vi "GetShortcut.vi"(8 "error in (no error)":errorcluster, 11 "separator item in":refnum<class "separator item.lvclass">) -> (0 "error out":errorcluster, 2 "shortcut":string, 3 "separator item out":refnum<class "separator item.lvclass">)   [LabVIEW 2009, in "separator item.lvclass"]
uses:
  separator item.lvclass
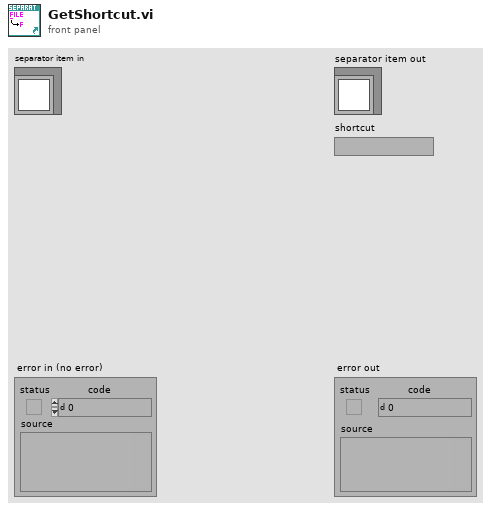
[diagram p1: front panel]
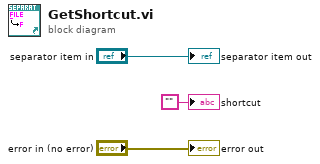
[diagram p0: block diagram]
diagram:
  "separator item out" <- "separator item in"
  "error out" <- "error in (no error)"
  "shortcut" <- ""
